vi "open.vi"(8 "error in (no error)":errorcluster caption="错误输入（无错误）", 11 "TCP_client 输入":refnum<class "TCP_client.lvclass">) -> (0 "error out":errorcluster caption="错误输出", 3 "TCP_client 输出":refnum<class "TCP_client.lvclass">)   [LabVIEW 2022 SP3, in "update.lvlib" / "TCP_client.lvclass"]
uses:
  TCP_client.lvclass
  TCP_client.lvclass/TCP_client.ctl
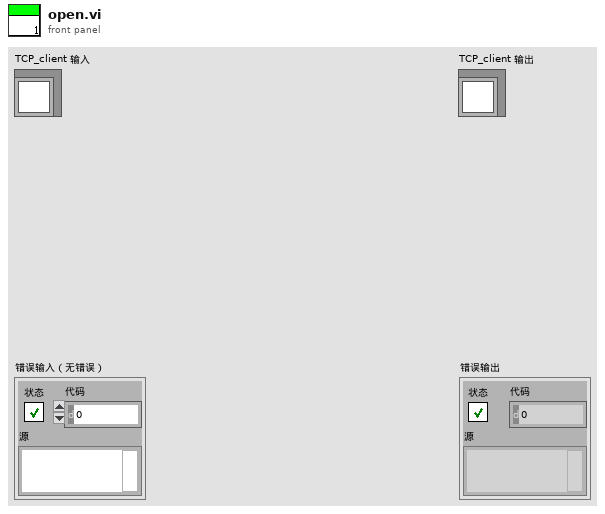
[diagram p1: front panel]
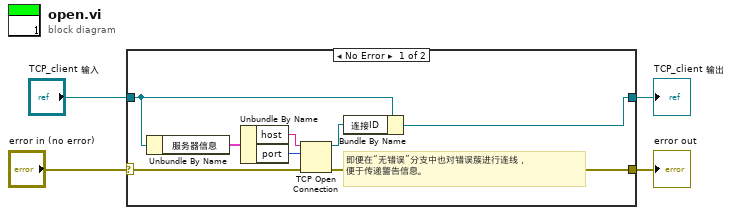
[diagram p0: block diagram]
diagram:
  n1 = case shown="No Error" "error in (no error)" {
    selector: "error in (no error)" -> [w6 w14]
    tunnel: [w5 w14] -> w3
    tunnel: [w8 w13] -> w1
    tunnel: "TCP_client 输入" -> [w9 w13]
    frame No Error {
      # "即便在“无错误”分支中也对错误簇进行连线，\n便于传递警告信息。"
      n2 = Unbundle By Name(w9) -> ("服务器信息"=w12:cluster{"host":string, "port":u16})
      n3 = Unbundle By Name(w12) -> ("host"=w11:string, "port"=w10:u16)
      n4 = TCP Open Connection(address=w11, remote port or service name=w10, error in (no error)=w6) -> (connection ID=w7:refnum<k5>, error out=w5:errorcluster)  [unwired: 2 in]
      n5 = Bundle By Name(cluster=w9, "连接ID"=w7) -> (w8:refnum<class "TCP_client.lvclass">)
    }
    frame Error {
    }
  }
  "error out" <- w3
  "TCP_client 输出" <- w1
